vi "String Trimming 1D.vi"(7 "Trimming Option":T1=enum."Trimg Empty and Sapce String" caption="Enum 3", 10 "1D String In":string[](array[string])) -> (2 "1D String Out":string[](array[string]))   [LabVIEW 2024]
uses:
  Typdef/String Trmming Option.ctl
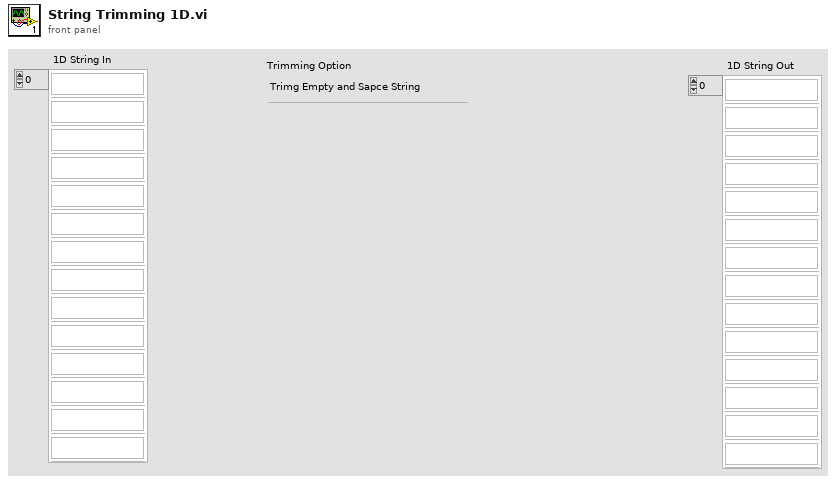
[diagram p1: front panel]
types:
  T1 = typedef "String Trmming Option.ctl" = enum16{"None", "Trim Empty String", "Trim Space String", "Trimg Empty and Sapce String"}
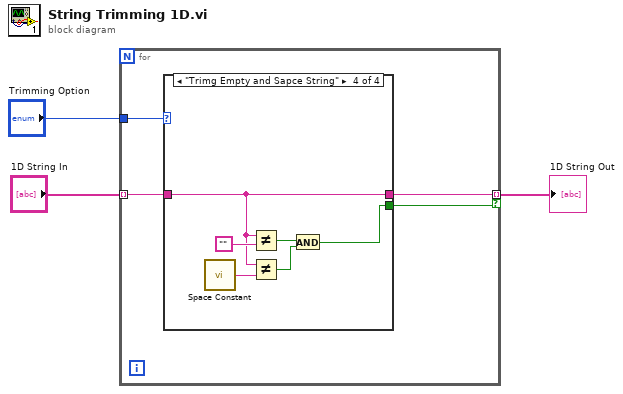
[diagram p0: block diagram]
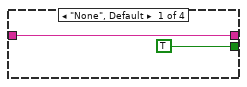
[diagram p2: hidden frame]
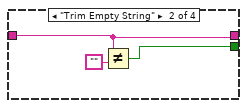
[diagram p3: hidden frame]
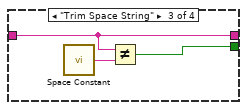
[diagram p4: hidden frame]
diagram:
  n1 = for {
    tunnel: "1D String In" -> [w6] mode=indexing
    tunnel: "Trimming Option" -> [w7]
    tunnel: [w5] -> w1 mode=indexing if=w4
    n2 = case shown="\"Trimg Empty and Sapce String\"" w7 {
      tunnel: w6 -> [w9 w10 w14 w19]
      tunnel: [w9 w10 w14 w19] -> w5
      tunnel: [TRUE w11 w15 w16] -> w4
      frame "None", Default {
      }
      frame "Trim Empty String" {
        n3 = Not Equal?(x=w10, y="") -> (x != y?=w11:bool)
      }
      frame "Trim Space String" {
        n4 = call <vilib>:"Space Constant.vi"() -> ("String"=w13:string)
        n5 = Not Equal?(x=w14, y=w13) -> (x != y?=w15:bool)
      }
      frame "Trimg Empty and Sapce String" {
        n6 = call <vilib>:"Space Constant.vi"() -> ("String"=w20:string)
        n7 = Not Equal?(x=w19, y="") -> (x != y?=w18:bool)
        n8 = Not Equal?(x=w19, y=w20) -> (x != y?=w17:bool)
        n9 = And(x=w18, y=w17) -> (x .and. y?=w16:bool)
      }
    }
  }
  "1D String Out" <- w1
